vi "SVT Fractional Octave Filtering.vi"   [LabVIEW 2017, in "SoundVib_Octave_2014 standard.lvlib"]
doc: "Performs fractional octave filtering on <B>scaled signal [EU]</B> in accordance with either the ANSI S1.11-2014 standard or the IEC 61260-1:2014 standard.\n\n \n\nYou can use this polymorphic VI to perform fractional octave filtering on a single channel or on N channels. The data type you wire to the <B>scaled signal [EU]</B> input determines the polymorphic instance to use."
uses:
  <vilib>/addons/Sound and Vibration/svt_Octave/SoundVib_Octave_2014 standard.lvlib
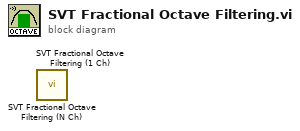
[diagram p0: block diagram]
diagram:
  n1 = call <vilib>:"SVT Fractional Octave Filtering (N Ch).vi"() -> ()  [unwired: 8 in, 4 out]
  n2 = call <vilib>:"SVT Fractional Octave Filtering (1 Ch).vi"() -> ()  [unwired: 8 in, 4 out]
